vi "Takeoff Aircraft.vi"(8 "Error In":errorcluster) -> (0 "Error Out":errorcluster)   [LabVIEW 2014]
uses:
  Controls/MAVLink Flight modes.ctl
  Aircraft Information/Sub VI/Get Aircraft Information.vi
  Waypoint Controller/FGV/Methods/Get Waypoint Transfer Status.vi
  Controls/Takeoff States.ctl
  Missions/FGVs/Virtual Waypoints/Methods/Get Virtual Waypoints.vi
  Application Support/Stop Button/SubVI/Get Stop Button Status.vi
  Missions/Controls/Waypoint Type.ctl
  Missions/Controls/Virtual Waypoint.ctl
  Aircraft Information/Sub VI/Selected Aircraft/SubVI/Get Selected Aircraft.vi
  Aircraft Information/Sub VI/Get Aircraft System Status.vi
  GUI Design/Buttons/Standard button.ctl
panel:
  out "Takeoff Status":string
  in  "Cancel":T1
  out "Upload Progress":dbl(slide) scale=0.0..100.0
  out "Takeoff Status":bool
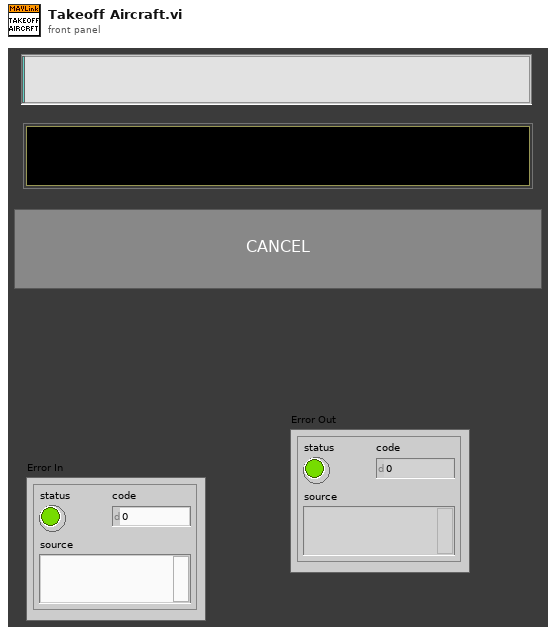
[diagram p1: front panel]
types:
  T1 = typedef "Standard button.ctl" = bool
  T2 = typedef "Takeoff States.ctl" = enum16{"Check if mission has changed", "Check waypoint heights", "Build and Upload New Mission", "Monitor Upload Status", "Set Aircraft Mode", "Arm Aircraft", "Launch Aircraft", "Launch Failure"}
  T3 = typedef "Virtual Waypoint.ctl" = cluster{"Waypoint Type":T4, "Lat":sgl, "Lon":sgl, "Altitude (m)":sgl, "Inspection Height (m)":sgl, "Circumnavigate Radius (m)":sgl, "Grid Waypoint?":bool, "Capture Photo":bool, "Speed (m/s)":sgl}
  T4 = typedef "Waypoint Type.ctl" = enum16{"PASS-THROUGH", "INSPECT", "CIRCUMNAVIGATE"}
  T5 = typedef "Drone Information.ctl" = cluster{"Aircraft ID":u8, "Tag ID":string, "System Status":string, "Base Mode":T6, "Armed/Disarmed":bool, "Battery Voltage":dbl, "Control Mode":T7, "Initialisation":u8, "Coms with aircraft good":bool, "Mode":string, "Mission Uploaded":bool}
  T6 = typedef "Base Mode.ctl" = cluster{"Custom Mode":bool, "Test Enabled":bool, "Autonomous Mode":bool, "Guided Mode":bool, "Stabilization Enabled":bool, "HIL Enabled":bool, "Manual Mode":bool, "Arm":bool}
  T7 = typedef "Aircraft Mode.ctl" = enum16{"Loiter", "Stabalise", "Failsafe", "Emergency Stop"}
  T8 = typedef "Aircraft Sensor Status Data.ctl" = cluster{"Sensor Status":T9, "CPU Load (%)":dbl, "Battery Voltage (V)":dbl, "Battery Current (A)":dbl, "Battery Remaining (%)":dbl, "Communication Drop Rate (%)":dbl, "Communication Errors (%)":dbl, "Status text":string}
  T9 = typedef "Sensor Status LED CLuster.ctl" = cluster{"3D Gyro":u32, "3D Accel":u32, "3D Mag":u32, "Abs. Pressure":u32, "Diff. Pressure":u32, "GPS":T10, "Optical Flow":u32, "Vision Position":u32, "Laser Position":u32, "External Ground Truth":u32, "Angular Rate Control":u32, "Attitude Stabilisation":u32, "Yaw Position":u32, "Z Altitude Control":u32, "XY Position Control":u32, "Motor Outputs":u32, "RC Receiver":u32, "3D Gyro 2":u32, "3D Accel 2":u32, "3D Mag 2":u32, "Geofence":u32, "AHRS":u32, "Terrain":u32}
  T10 = typedef "Status LED.ctl" = u32
  T11 = typedef "MAVLink Flight modes.ctl" = enum32{"STABILISE", "ACRO", "ALT HOLD", "AUTO", "GUIDED", "LOITER", "RTL", "CIRCLE", "UNKNOWN1", "LAND", "OF LOITER", "DRIFT", "UNKNOWN2", "SPORT", "FLIP", "AUTO TUNE", "POS HOLD", "BRAKE"}
  T12 = typedef "Waypoint Transfer Status.ctl" = cluster{"Upload Complete":bool, "Transfer Progress (Upload)":dbl, "Download Complete":bool, "Transfer Progress (Download)":dbl}
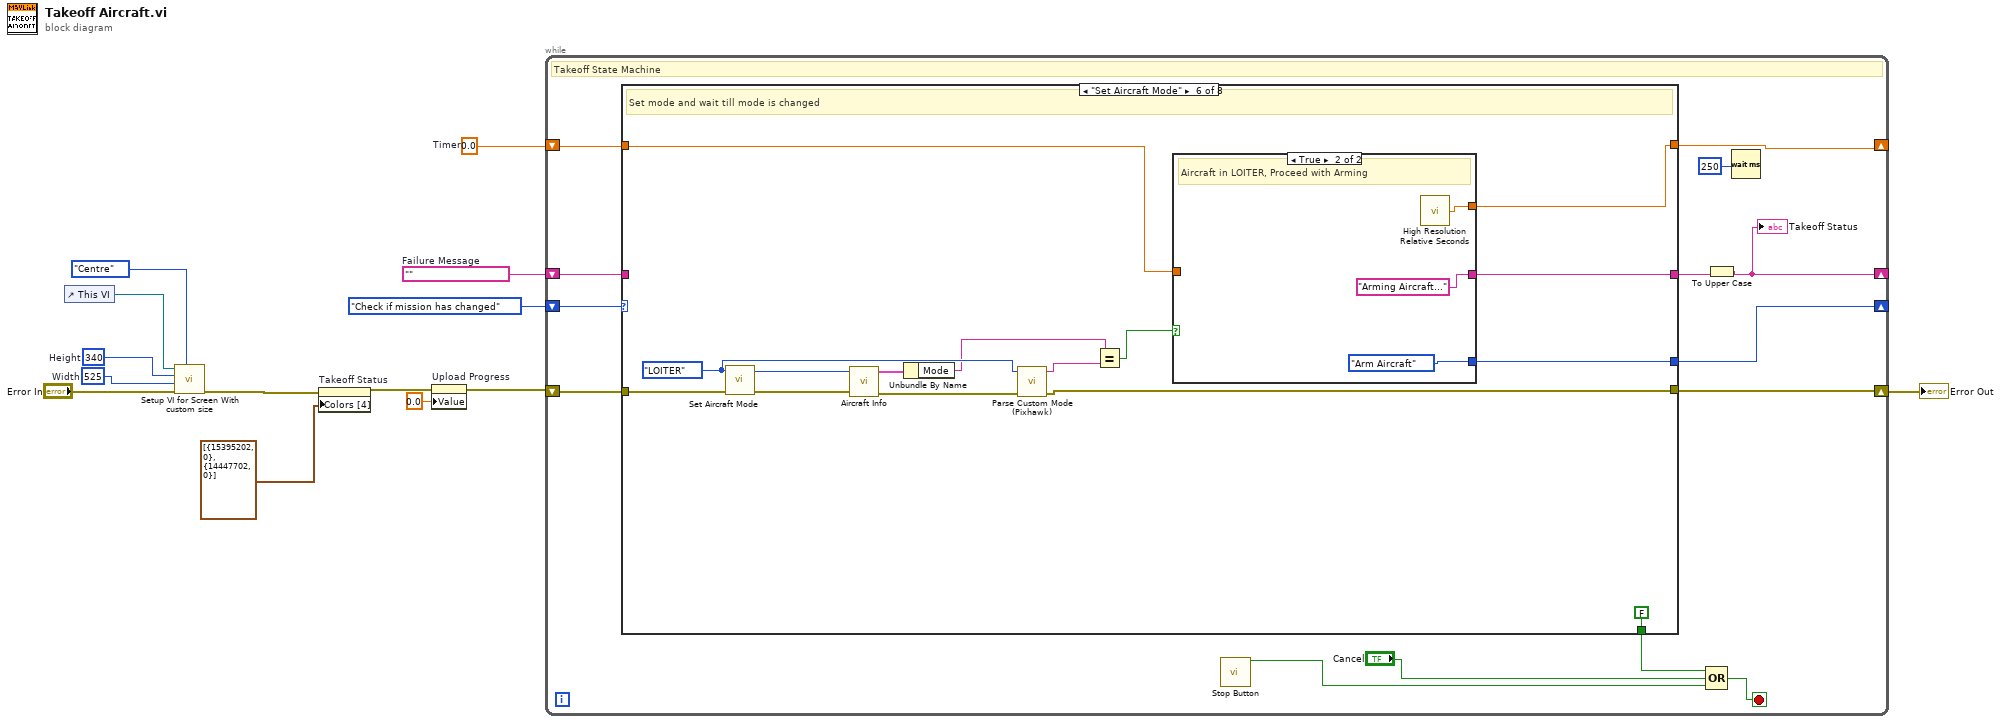
[diagram p0: block diagram]
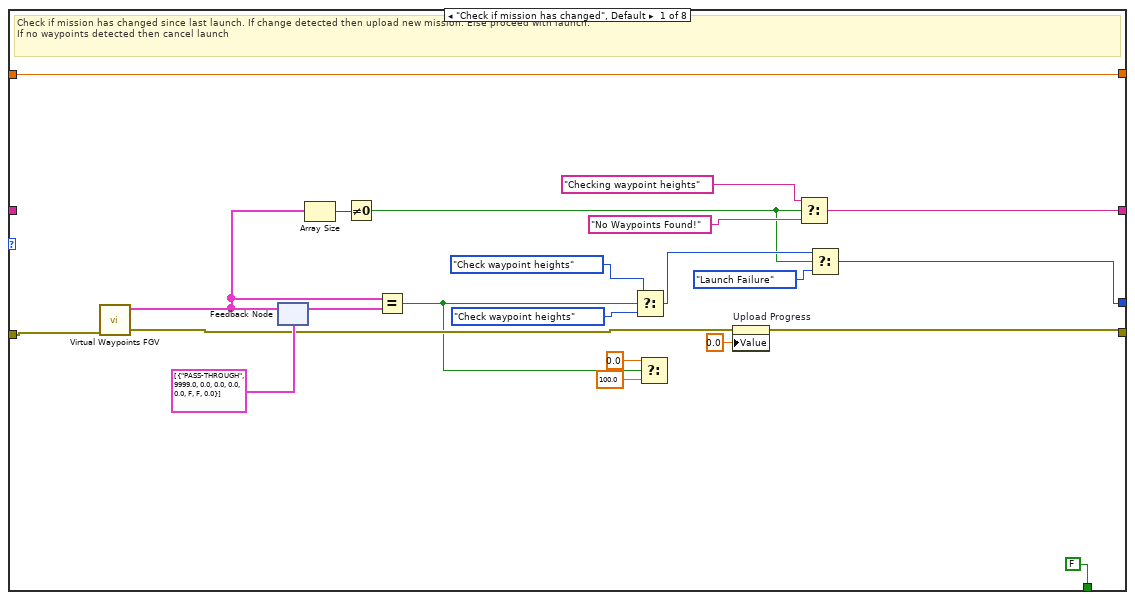
[diagram p2: hidden frame]
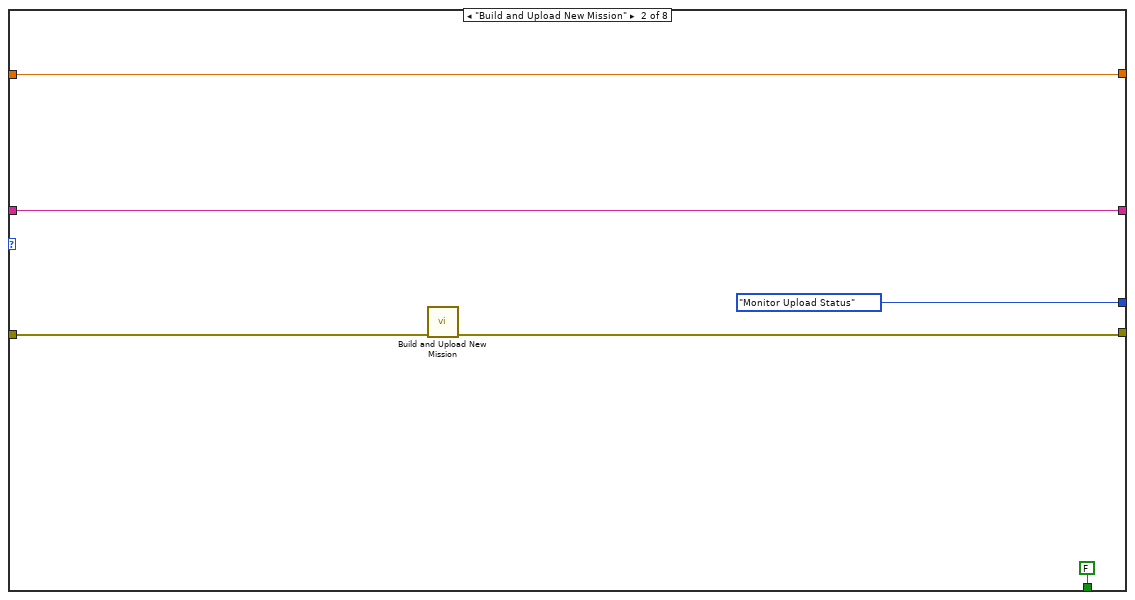
[diagram p3: hidden frame]
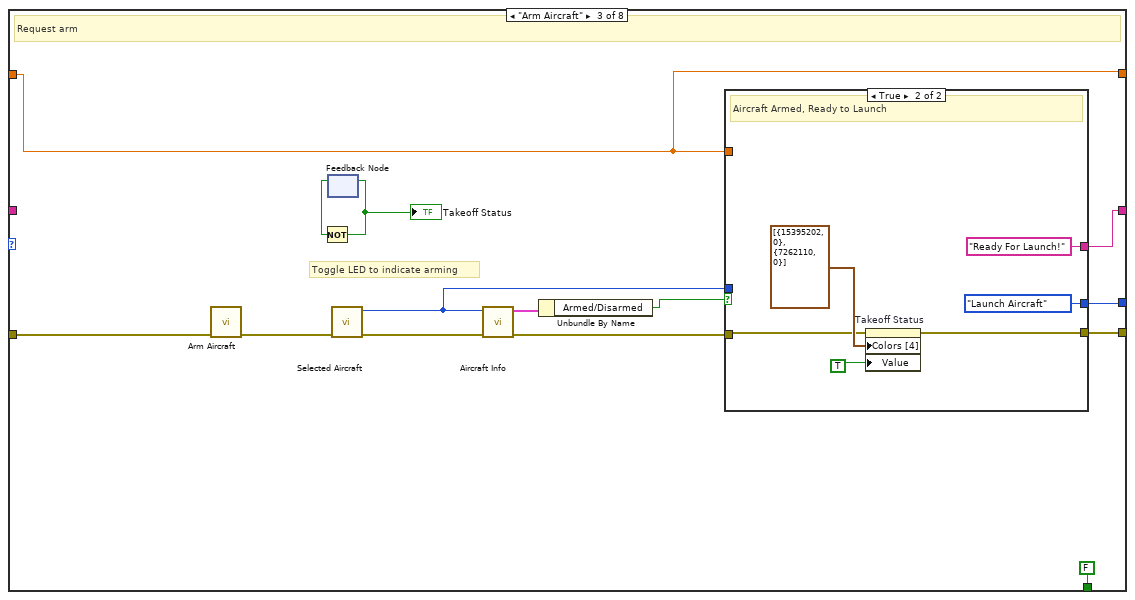
[diagram p4: hidden frame]
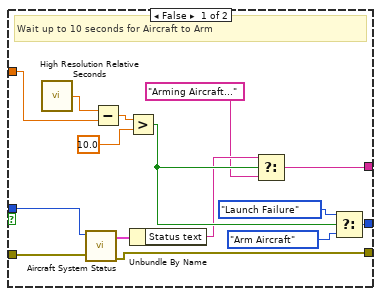
[diagram p5: hidden frame]
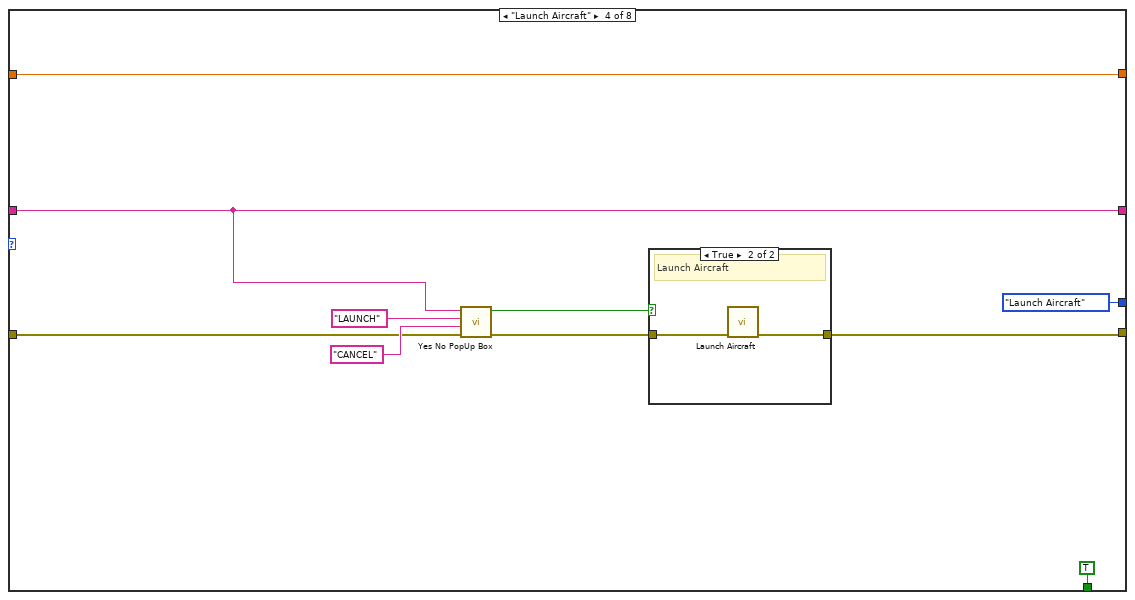
[diagram p6: hidden frame]
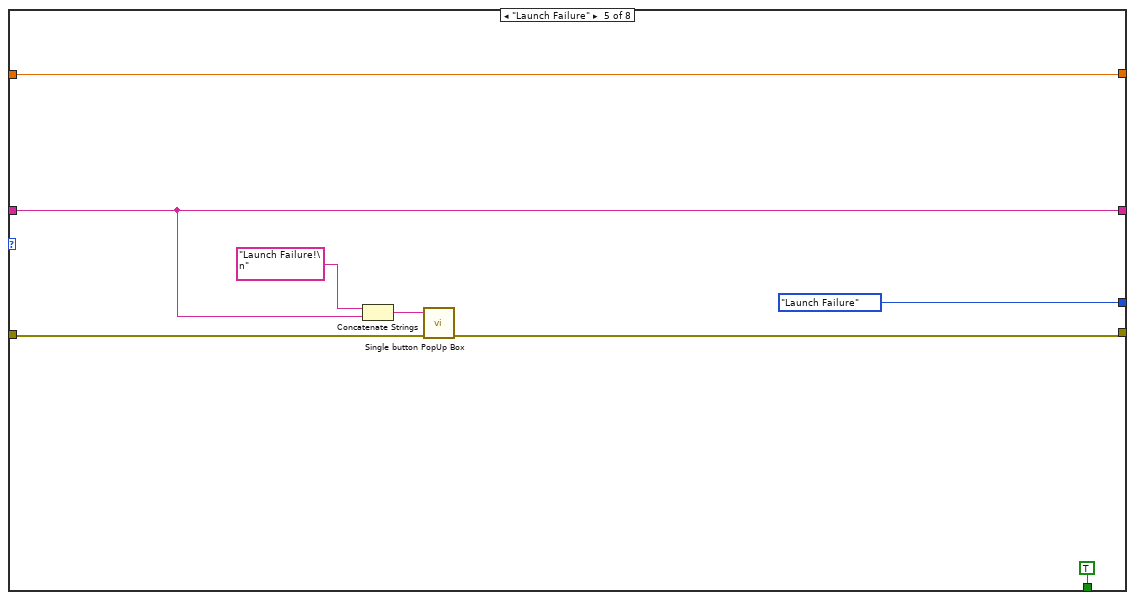
[diagram p8: hidden frame]
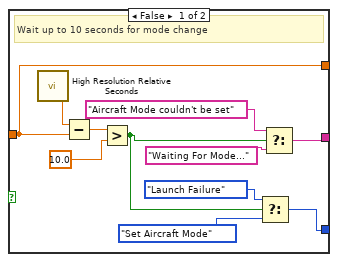
[diagram p9: hidden frame]
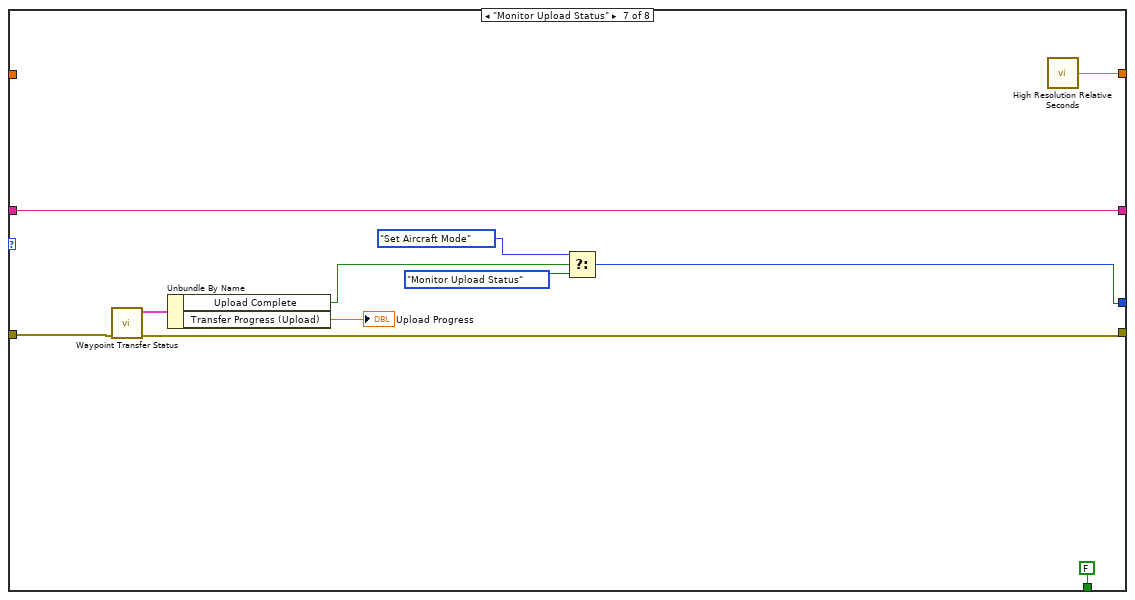
[diagram p10: hidden frame]
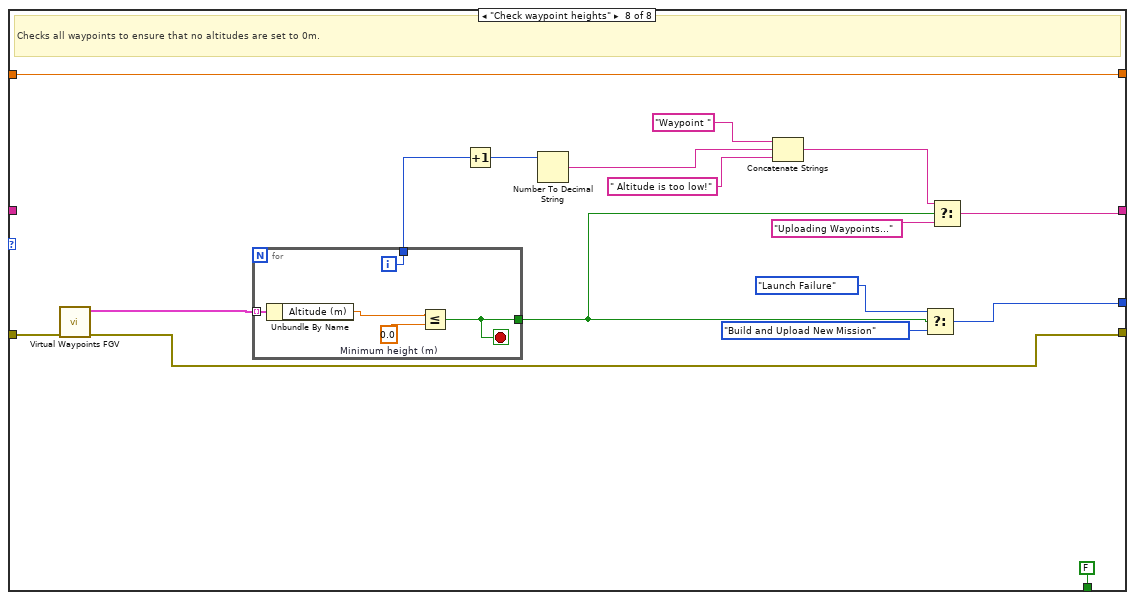
[diagram p11: hidden frame]
diagram:
  w5 = 0.0  # Timer
  w6 = ""  # Failure Message
  w10 = i16 525  # Width
  w11 = i16 340  # Height
  n1 = control-ref of="This VI"() -> (w13:refnum<vi>)
  n2 = call "Setup VI for Screen With custom size.vi"("Position"=enum16{"Top Left", "Centre"}."Centre", "Error In"="Error In", "Width"=w10, "Height"=w11, "This VI"=w13) -> ("Error Out"=w9:errorcluster)  [unwired: 5 in, 1 out]
  n3 = property on="Takeoff Status" class="Bool (strict)"(error in=w9, "Colors [4]"=cluster{u32, u32}[] [{15395202, 0}, {14447702, 0}]) -> (error out=w2:errorcluster)  [unwired: 1 in, 1 out]
  n4 = property on="Upload Progress" class="Slide (strict)"(error in=w2, "Value"=0.0 ("Upload Progress")) -> (error out=w3:errorcluster)  [unwired: 1 in, 1 out]
  n5 = while {
    shift-right: [w21] -> _
    shift-left: Takeoff_States."Check if mission has changed" ("Takeoff States") -> [w28]
    shift-right: [w15] -> _
    shift-left: w6 -> [w22]
    shift-right: [w20] -> w4
    shift-left: w3 -> [w27]
    shift-right: [w17] -> _
    shift-left: w5 -> [w18]
    stop <- w23 stop-if-true
    # "Takeoff State Machine"
    n6 = case shown="\"Set Aircraft Mode\"" w28 {
      tunnel: w27 -> [w50 w56 w70 w99 w109 w126 w152 w168]
      tunnel: [FALSE ("value") FALSE ("value") FALSE ("value") TRUE ("value") TRUE ("value") FALSE ("value") FALSE ("value") FALSE ("value")] -> w24
      tunnel: w22 -> [_ w54 _ w93 w110 _ w144 _]
      tunnel: [w36 w54 w62 w93 w110 w116 w144 w161] -> w16
      tunnel: [w31 Takeoff_States."Monitor Upload Status" ("Takeoff States") w61 Takeoff_States."Launch Aircraft" ("f") Takeoff_States."Launch Failure" ("f") w117 w146 w157] -> w21
      tunnel: [w44 w55 w63 w96 w108 w115 w145 w156] -> w20
      tunnel: w18 -> [w30 w51 w65 w92 w105 w114 _ w169]
      tunnel: [w30 w51 w65 w92 w105 w113 w143 w169] -> w17
      frame "Check if mission has changed", Default {
        # "Check if mission has changed since last launch. If change detected then upload new mission. Else proceed with launch. \nIf no waypoints detected then cancel launch"
        n7 = call-poly "Virtual Waypoints FGV.vi"("Error In"=w50) -> ("Error Out"=w43:errorcluster, "Virtual Waypoints Out"=w38:T3[])  [unwired: 9 in]
        n8 = feedback-in #1(w38) -> ()
        n9 = feedback #1(T3[] [{"Waypoint Type"=enum."PASS-THROUGH", "Lat"=9999.0, "Lon"=0.0, "Altitude (m)"=0.0, "Inspection Height (m)"=0.0, "Circumnavigate Radius (m)"=0.0, "Grid Waypoint?"=FALSE, "Capture Photo"=FALSE, "Speed (m/s)"=0.0}] ("Virtual Waypoints Out")) -> (w47:T3[])
        n10 = Array Size(array=w38) -> (size(s)=w37:i32)
        n11 = Not Equal To 0?(x=w37) -> (x != 0?=w33:bool)
        n12 = Equal?(x=w38, y=w47) -> (x = y?=w42:bool)
        n13 = Select(t=Takeoff_States."Check waypoint heights" ("Takeoff States"), s=w42, f=Takeoff_States."Check waypoint heights" ("Takeoff States")) -> (s? t:f=w34:T2)
        n14 = Select(t=0.0, s=w42, f=100.0) -> ()  [unwired: 1 out]
        n15 = property on="Upload Progress" class="Slide (strict)"(error in=w43, "Value"=0.0 ("Upload Progress")) -> (error out=w44:errorcluster)  [unwired: 1 in, 1 out]
        n16 = Select(t="Checking waypoint heights" ("Failure Message"), s=w33, f="No Waypoints Found!") -> (s? t:f=w36:string)
        n17 = Select(t=w34, s=w33, f=Takeoff_States."Launch Failure") -> (s? t:f=w31:T2)
      }
      frame "Build and Upload New Mission" {
        n18 = call "Build and Upload New Mission.vi"("Error In"=w56) -> ("Error Out"=w55:errorcluster)  [unwired: 10 in]
      }
      frame "Arm Aircraft" {
        # "Toggle LED to indicate arming"
        # "Request arm"
        n19 = call "Arm Aircraft.vi"("Error In"=w70) -> ("error out"=w69:errorcluster)  [unwired: 9 in, 1 out]
        n20 = feedback #2() -> (w60:bool)  [unwired: 1 in]
        n21 = Not(x=w60) -> (.not. x?=w59:bool)
        "Takeoff Status" <- w59
        n22 = feedback-in #2(w59) -> ()
        n23 = call-poly "Selected Aircraft.vi"("Error In"=w69) -> ("Error Out"=w68:errorcluster, "Selected Aircraft ID Out"=w57:u8)  [unwired: 9 in]
        n24 = call-poly "Aircraft Info.vi"("Error In"=w68, "Aircraft ID"=w57) -> ("Error Out"=w64:errorcluster, "Aircraft Information Out"=w67:T5)  [unwired: 8 in]
        n25 = Unbundle By Name(w67) -> ("Armed/Disarmed"=w66:bool)
        n26 = case shown="True" w66 {
          tunnel: w65 -> [w82 _]
          tunnel: w64 -> [w81 w86]
          tunnel: [w77 w87] -> w63
          tunnel: [w75 "Ready For Launch!" ("f")] -> w62
          tunnel: [w72 Takeoff_States."Launch Aircraft" ("Takeoff States")] -> w61
          tunnel: w57 -> [w71 _]
          frame False {
            # "Wait up to 10 seconds for Aircraft to Arm"
            n27 = call <vilib>:"High Resolution Relative Seconds.vi"() -> ("relative seconds"=w85:dbl)
            n28 = call-poly "Aircraft System Status.vi"("Error In"=w81, "Aircraft ID"=w71) -> ("Error Out"=w77:errorcluster, "System Status Out"=w80:T8)  [unwired: 8 in]
            n29 = Subtract(x=w85, y=w82) -> (x-y=w84:dbl)
            n30 = Greater?(x=w84, y=10.0) -> (0:w79:bool)
            n31 = Unbundle By Name(w80) -> ("Status text"=w78:string)
            n32 = Select(t=w78, s=w79, f="Arming Aircraft...") -> (s? t:f=w75:string)
            n33 = Select(t=Takeoff_States."Launch Failure" ("Takeoff States"), s=w79, f=Takeoff_States."Arm Aircraft" ("Takeoff States")) -> (s? t:f=w72:T2)
          }
          frame True {
            # "Aircraft Armed, Ready to Launch"
            n34 = property on="Takeoff Status" class="Bool (strict)"(error in=w86, "Colors [4]"=cluster{u32, u32}[] [{15395202, 0}, {7262110, 0}], "Value"=TRUE ("Takeoff Status")) -> (error out=w87:errorcluster)  [unwired: 1 in, 1 out]
          }
        }
      }
      frame "Launch Aircraft" {
        n35 = call "Yes No PopUp Box.vi"("Error In"=w99, "Cancel Button Text"="CANCEL", "Done Button text"="LAUNCH", "Input Message"=w93) -> ("Error Out"=w97:errorcluster, "User DOne"=w98:bool)  [unwired: 6 in]
        n36 = case shown="True" w98 {
          tunnel: w97 -> [w102 w104]
          tunnel: [w102 w103] -> w96
          frame False {
            # "User Cancelled Launch"
          }
          frame True {
            # "Launch Aircraft"
            n37 = call "Launch Aircraft.vi"("Error In"=w104) -> ("error out"=w103:errorcluster)  [unwired: 10 in]
          }
        }
      }
      frame "Launch Failure" {
        n38 = Concatenate Strings("Launch Failure!\n" ("message"), w110) -> (w111:string)
        n39 = call "Single button PopUp Box.vi"("Error In"=w109, "Input Message"=w111) -> ("Error Out"=w108:errorcluster)  [unwired: 8 in, 1 out]
      }
      frame "Set Aircraft Mode" {
        w122 = MAVLink_Flight_modes."LOITER" ("Aircraft Mode")
        # "Set mode and wait till mode is changed"
        n40 = call "Set Aircraft Mode.vi"("Error In"=w126, "Aircraft Mode"=w122) -> ("error out"=w125:errorcluster, "Selected Aircraft ID Out"=w124:u8)  [unwired: 8 in]
        n41 = call-poly "Aircraft Info.vi"("Error In"=w125, "Aircraft ID"=w124) -> ("Error Out"=w123:errorcluster, "Aircraft Information Out"=w120:T5)  [unwired: 8 in]
        n42 = Unbundle By Name(w120) -> ("Mode"=w119:string)
        n43 = call "Parse Custom Mode (Pixhawk).vi"("Error In"=w123, "custom mode"=w122) -> ("Error Out"=w115:errorcluster, "Custom Mode"=w121:string)  [unwired: 8 in]
        n44 = Equal?(x=w119, y=w121) -> (x = y?=w118:bool)
        n45 = case shown="True" w118 {
          tunnel: [w136 Takeoff_States."Arm Aircraft" ("f")] -> w117
          tunnel: [w134 "Arming Aircraft..." ("Failure Message")] -> w116
          tunnel: w114 -> [w128 _]
          tunnel: [w128 w139] -> w113
          frame False {
            # "Wait up to 10 seconds for mode change"
            n46 = call <vilib>:"High Resolution Relative Seconds.vi"() -> ("relative seconds"=w132:dbl)
            n47 = Subtract(x=w132, y=w128) -> (x-y=w131:dbl)
            n48 = Greater?(x=w131, y=10.0) -> (0:w129:bool)
            n49 = Select(t=Takeoff_States."Launch Failure" ("Takeoff States"), s=w129, f=Takeoff_States."Set Aircraft Mode") -> (s? t:f=w136:T2)
            n50 = Select(t="Aircraft Mode couldn't be set", s=w129, f="Waiting For Mode..." ("Mode")) -> (s? t:f=w134:string)
          }
          frame True {
            # "Aircraft in LOITER, Proceed with Arming"
            n51 = call <vilib>:"High Resolution Relative Seconds.vi"() -> ("relative seconds"=w139:dbl)
          }
        }
      }
      frame "Monitor Upload Status" {
        n52 = call-poly "Waypoint Transfer Status.vi"("Error In"=w152) -> ("Error Out"=w145:errorcluster, "Waypoint Transfer Status Out"=w151:T12)  [unwired: 9 in]
        n53 = Unbundle By Name(w151) -> ("Upload Complete"=w149:bool, "Transfer Progress (Upload)"=→"Upload Progress":dbl)
        n54 = Select(t=Takeoff_States."Set Aircraft Mode" ("Takeoff States"), s=w149, f=Takeoff_States."Monitor Upload Status") -> (s? t:f=w146:T2)
        n55 = call <vilib>:"High Resolution Relative Seconds.vi"() -> ("relative seconds"=w143:dbl)
      }
      frame "Check waypoint heights" {
        # "Checks all waypoints to ensure that no altitudes are set to 0m."
        n56 = call-poly "Virtual Waypoints FGV.vi"("Error In"=w168) -> ("Error Out"=w156:errorcluster, "Virtual Waypoints Out"=w167:T3[])  [unwired: 9 in]
        n57 = for {
          tunnel: w167 -> [w174] mode=indexing
          tunnel: [w171] -> w159
          tunnel: [w170] -> w154
          i -> [w170]
          stop <- w171 stop-if-true
          w172 = sgl 0.0  # Minimum height (m)
          n58 = Unbundle By Name(w174) -> ("Altitude (m)"=w173:sgl)
          n59 = Less Or Equal?(x=w173, y=w172) -> (x <= y?=w171:bool)
        }
        n60 = Increment(x=w154) -> (x+1=w153:i32)
        n61 = Number To Decimal String(number=w153) -> (decimal integer string=w165:string)  [unwired: 1 in]
        n62 = Concatenate Strings("Waypoint " ("string"), w165, " Altitude is too low!" ("string")) -> (w162:string)
        n63 = Select(t=Takeoff_States."Launch Failure" ("f"), s=w159, f=Takeoff_States."Build and Upload New Mission") -> (s? t:f=w157:T2)
        n64 = Select(t=w162, s=w159, f="Uploading Waypoints..." ("Failure Message")) -> (s? t:f=w161:string)
      }
    }
    n65 = call-poly "Stop Button.vi"() -> ("Stop ButtonOut"=w25:bool)  [unwired: 10 in, 1 out]
    n66 = Compound Arithmetic op=OR(w24, "Cancel", w25) -> (w23:T1)
    n67 = To Upper Case(1:w16) -> (0:w15:string)
    "Takeoff Status" <- w15
    n68 = Wait (ms)(milliseconds to wait=u32 250) -> ()  [unwired: 1 out]
  }
  "Error Out" <- w4
